vi "view.vi"(8 "error in (no error)":errorcluster, 11 "Value in":refnum<class "Value.lvclass">) -> (0 "error out":errorcluster, 1 "grad":T3, 2 "Value":T3, 3 "Value out":refnum<class "Value.lvclass">, 6 "label":T2)   [LabVIEW 2023, in "LabGRAD.lvlib" / "Value.lvclass"]
uses:
  Value.lvclass
  UiObjects/numeric value control.ctl
  UiObjects/string control.ctl
  operation.ctl
  Value.lvclass/Value.ctl
  UiObjects/UiObjects.lvclass
panel:
  out "Other":variant
  out "Previous":variant
  out "operation":T1=enum."add"
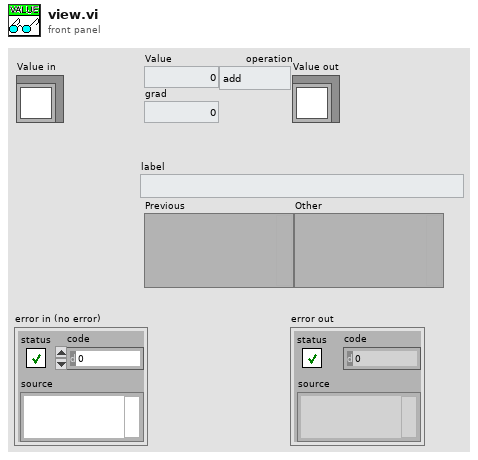
[diagram p1: front panel]
types:
  T1 = typedef "LabGRAD.lvlib/Value.lvclass/operation.ctl" = enum16{"nop", "add", "subtract", "power", "multiply", "divide", "tanh"}
  T2 = typedef "UiObjects.lvlib/UiObjects.lvclass/string control.ctl" = string
  T3 = typedef "UiObjects.lvlib/UiObjects.lvclass/numeric value control.ctl" = dbl
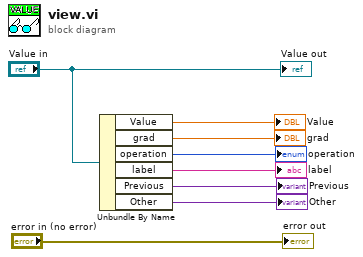
[diagram p0: block diagram]
diagram:
  n1 = Unbundle By Name("Value in") -> ("Value"=→"Value":T3, "grad"=→"grad":T3, "operation"=→"operation":T1, "label"=→"label":T2, "Previous"=→"Previous":variant, "Other"=→"Other":variant)
  "error out" <- "error in (no error)"
  "Value out" <- "Value in"
